vi "Project Omega.vi"() -> ()   [LabVIEW 2020]
uses:
  <vilib>/DAQmx/read.llb/DAQmx Read (Analog 2D DBL NChan NSamp).vi
  <vilib>/DAQmx/create/channels.llb/DAQmx Create Channel (AI-Voltage-Basic).vi
  <vilib>/DAQmx/create/channels.llb/DAQmx Create Channel (AI-Voltage-Custom with Excitation).vi
  <vilib>/DAQmx/configure/timing.llb/DAQmx Timing (Sample Clock).vi
  <vilib>/DAQmx/miscellaneous.llb/DAQmx Fill In Error Info.vi
  <vilib>/Analysis/NI_AALPro.lvlib
panel:
  in  "Path":path
  in  "STOP":bool
  out "Displacement(mm)":dbl[](array[numeric])
  out "Period of Vibration (T)":dbl
  out "Natural Frequency f(n)":dbl
  out "Circular Natural frequency w(n)":dbl
  out "Mass of the spring system(lbm)":dbl
  out "Displacement":dbl
  in  "Displacement offset":dbl
  in  "Load offset":dbl
  out "Force Value (lbf)":dbl
  out "Stiffness of spring(k)":dbl
  out "Load vs Displacement":cluster{dbl[], dbl[]}(graph)
  out "Load vs Time":cluster{dbl[], dbl[]}(graph)
  out "Displacement vs Time":cluster{dbl[], dbl[]}(graph)
  in  "DAQ Rate(Hz)":dbl
  in  "Time to acquire Data(s)":dbl
  in  "Load description":string="Pounds - lbf"
  in  "Displacement custom scale":tag
  in  "Displacement DAQ Channel":tag
  in  "Displacement  Description":string="Positon- inches"
  in  "Load Transducer Scale:":tag
  in  "Load DAQ Channel":tag
  # "DAQ Input"
  # "Results"
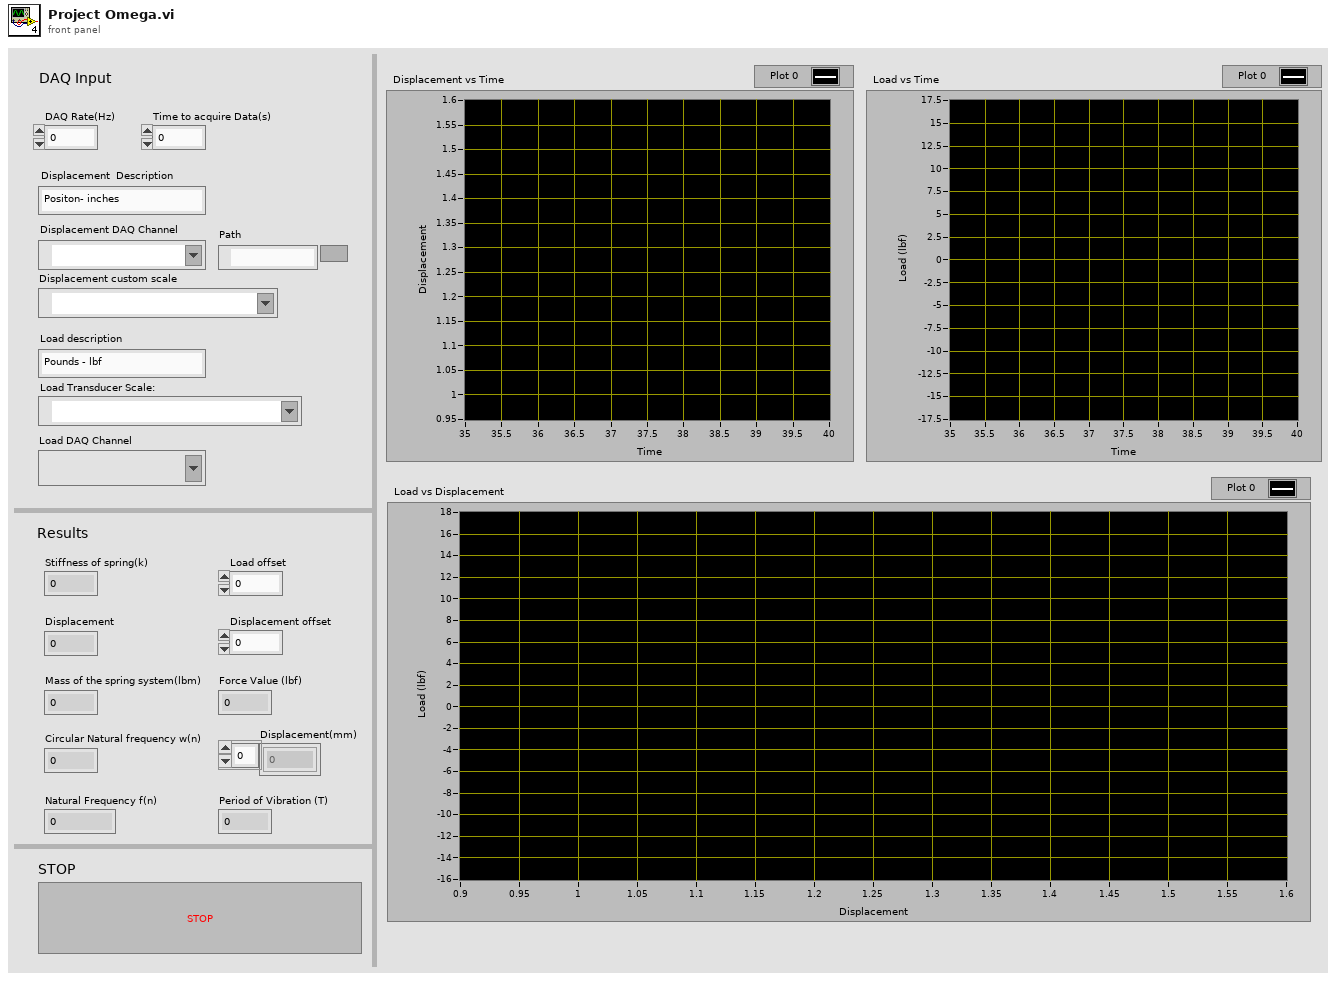
[diagram p1: front panel]
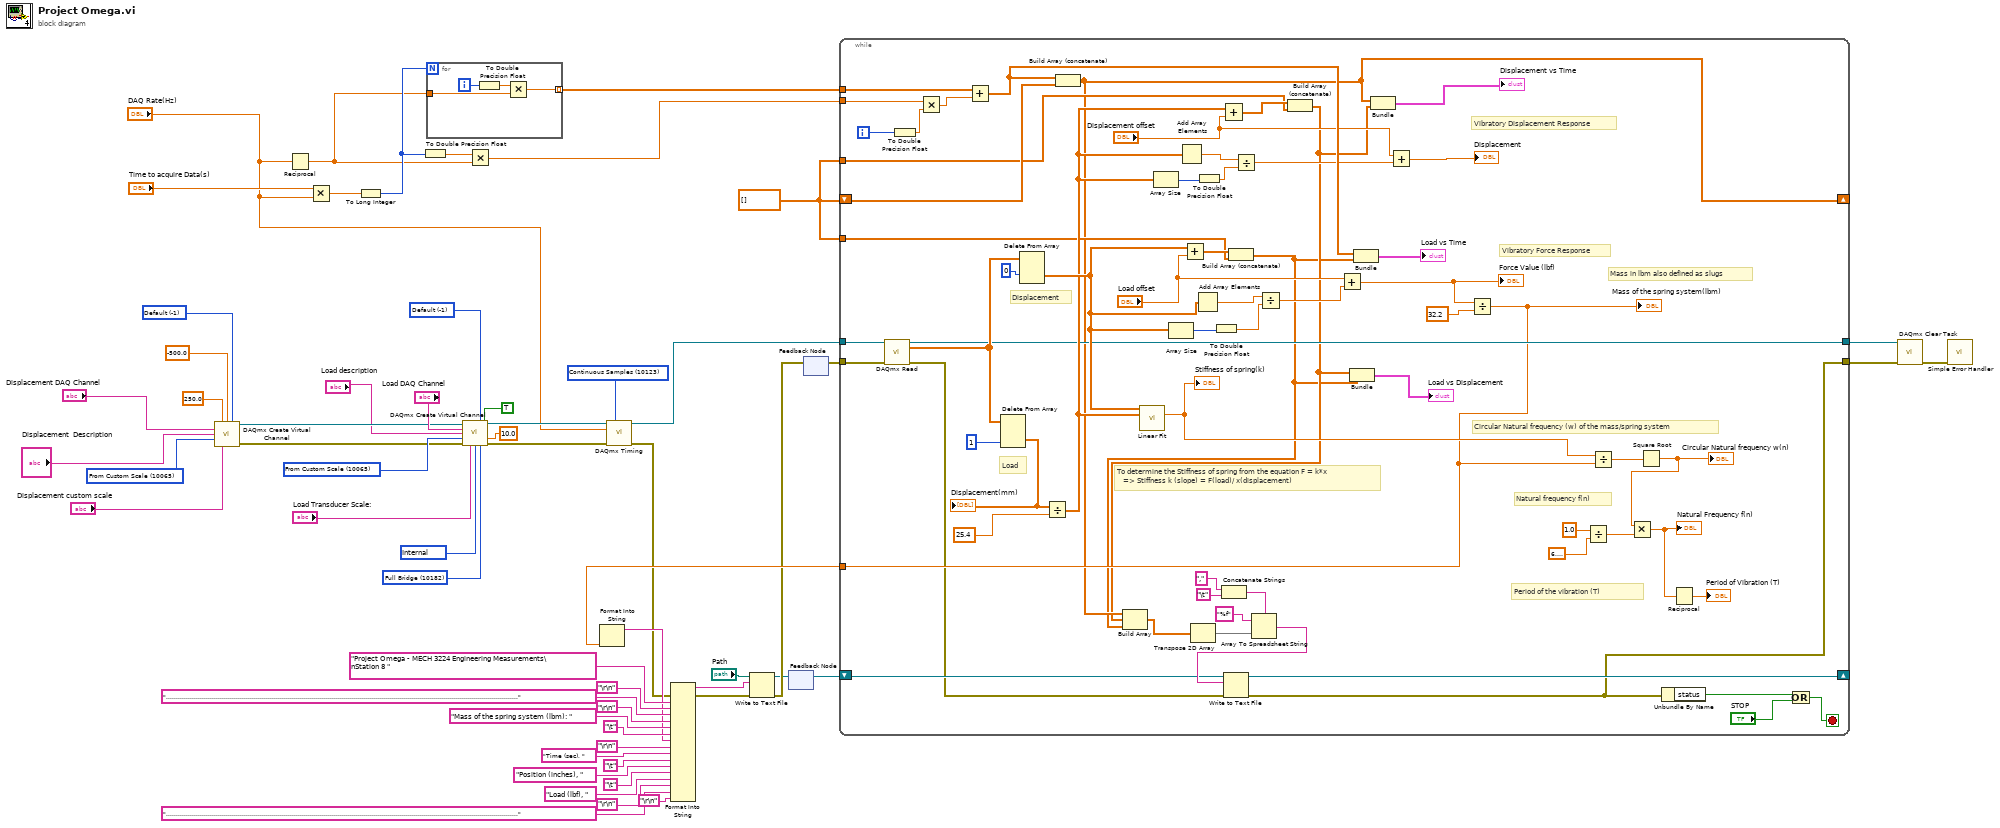
[diagram p0: block diagram]
diagram:
  w3 = dbl[] []
  w43 = 10065 items=["Volts"=10348, "From Custom Scale"=10065] ("units")
  w45 = -1 items=["Default"=-1, "RSE"=10083, "NRSE"=10078, "Differential"=10106, "Pseudodifferential"=12529] ("input terminal configuration")
  w39 = 10182 items=["Full Bridge"=10182, "Half Bridge"=10187, "Quarter Bridge"=10270, "No Bridge"=10228] ("bridge configuration")
  w53 = 10200 items=["Internal"=10200, "External"=10167, "None"=10230] ("voltage excitation source")
  w41 = 10123 items=["Finite Samples"=10178, "Continuous Samples"=10123, "Hardware Timed Single Point"=12522] ("sample mode")
  w55 = 10065 items=["Volts"=10348, "From Custom Scale"=10065] ("units")
  w57 = -1 items=["Default"=-1, "RSE"=10083, "NRSE"=10078, "Differential"=10106, "Pseudodifferential"=12529] ("input terminal configuration")
  n1 = call-poly <vilib>:"DAQmx Create Virtual Channel.vi"("maximum value"=250.0, "minimum value"=-500.0, "input terminal configuration"=w45, "physical channels"="Displacement DAQ Channel", "name to assign"="Displacement  Description", "units"=w43, "custom scale name"="Displacement custom scale") -> ("task out"=w51:refnum<k21>, "error out"=w40:errorcluster)  [unwired: 7 in]
  n2 = Reciprocal(x="DAQ Rate(Hz)") -> (1/x=w34:dbl)
  n3 = Multiply(x="Time to acquire Data(s)", y="DAQ Rate(Hz)") -> (x*y=w37:dbl)
  n4 = To Long Integer(number=w37) -> (32bit integer=w35:i32)
  n5 = To Double Precision Float(number=w35) -> (double precision float=w36:dbl)
  n6 = for {
    N: w35 -> [_]
    tunnel: w34 -> [w61]
    tunnel: [w60] -> w30 mode=indexing
    i -> [w63]
    n7 = To Double Precision Float(number=w63) -> (double precision float=w62:dbl)
    n8 = Multiply(x=w62, y=w61) -> (x*y=w60:dbl)
  }
  n9 = call-poly <vilib>:"DAQmx Create Virtual Channel.vi"("task in"=w51, "input terminal configuration"=w57, "physical channels"="Load DAQ Channel", "use excitation for scaling"=TRUE, "name to assign"="Load description", "units"=w55, "voltage excitation value"=10.0, "error in"=w40, "custom scale name"="Load Transducer Scale:", "voltage excitation source"=w53, "bridge configuration"=w39) -> ("task out"=w58:refnum<k21>, "error out"=w59:errorcluster)  [unwired: 3 in]
  n10 = Multiply(x=w36, y=w34) -> (x*y=w31:dbl)
  n11 = call-poly <vilib>:"DAQmx Timing.vi"("task/channels in"=w58, "sample mode"=w41, "rate"="DAQ Rate(Hz)", "error in"=w59) -> ("task out"=w32:refnum<k21>, "error out"=w8:errorcluster)  [unwired: 10 in]
  n12 = feedback #1() -> (w4:refnum<file>)  [unwired: 1 in]
  n13 = feedback #2() -> (w6:errorcluster)  [unwired: 1 in]
  n14 = while {
    tunnel: w32 -> [w89]
    tunnel: w31 -> [w87]
    tunnel: w30 -> [w86]
    tunnel: [w84] -> w29
    tunnel: [w83] -> w22
    tunnel: w6 -> [w82]
    shift-right: [w67] -> _
    shift-left: w4 -> [w68]
    tunnel: w3 -> [w81]
    shift-right: [w71] -> _
    shift-left: w3 -> [w80]
    tunnel: w3 -> [w79]
    tunnel: [w64] -> w1
    i -> [w88]
    stop <- w90 stop-if-true
    # "Period of the vibration (T)"
    # "Natural frequency f(n)"
    # "Circular Natural frequency (w) of the mass/spring system"
    # "Vibratory Displacement Response"
    # "Vibratory Force Response"
    # "Mass in lbm also defined as slugs"
    # "To determine the Stiffness of spring from the equation F = k*x\n   => Stiffness k (slope) = F(load)/ x(displacement)"
    # "Load"
    # "Displacement"
    n15 = call-poly <vilib>:"DAQmx Read.vi"("task/channels in"=w89, "error in"=w82) -> ("task out"=w84:refnum<k21>, "data"=w126:dbl[][], "error out"=w65:errorcluster)  [unwired: 11 in]
    n16 = To Double Precision Float(number=w88) -> (double precision float=w123:dbl)
    n17 = Multiply(x=w87, y=w123) -> (x*y=w122:dbl)
    n18 = Add(x=w86, y=w122) -> (x+y=w121:dbl[])
    n19 = Delete From Array(array=w126, index (row)=1) -> (deleted portion=w94:dbl[])  [unwired: 2 in, 1 out]
    "Displacement(mm)" <- w94
    n20 = Delete From Array(array=w126, index (row)=0 ("disabled index (col)")) -> (deleted portion=w115:dbl[])  [unwired: 2 in, 1 out]
    n21 = Divide(x=w94, y=25.4 ("Waveform")) -> (x/y=w92:dbl[])
    n22 = Build Array (concatenate)(w121, w80) -> (w71:dbl[])
    n23 = call <vilib>:"Linear Fit.vi"("Y"=w115, "X"=w92) -> ("slope"=w96:dbl)  [unwired: 9 in, 4 out]
    "Stiffness of spring(k)" <- w96
    n24 = Array Size(array=w92) -> (size(s)=w111:i32)
    n25 = Array Size(array=w115) -> (size(s)=w116:i32)
    n26 = Add Array Elements(numeric array=w92) -> (sum=w113:dbl)
    n27 = Add(x=w115, y="Load offset") -> (x+y=w120:dbl[])
    n28 = Add Array Elements(numeric array=w115) -> (sum=w118:dbl)
    n29 = To Double Precision Float(number=w111) -> (double precision float=w112:dbl)
    n30 = To Double Precision Float(number=w116) -> (double precision float=w117:dbl)
    n31 = Add(x=w92, y="Displacement offset") -> (x+y=w110:dbl[])
    n32 = Concatenate Strings("," ("delimiter (Tab)"), "\t") -> (w73:string)
    n33 = Build Array (concatenate)(w120, w81) -> (w69:dbl[])
    n34 = Divide(x=w113, y=w112) -> (x/y=w109:dbl)
    n35 = Divide(x=w118, y=w117) -> (x/y=w114:dbl)
    n36 = Build Array (concatenate)(w110, w79) -> (w70:dbl[])
    n37 = Build Array(w71, w70, w69) -> (w78:dbl[][])
    n38 = Transpose 2D Array(2D array=w78) -> (transposed array=w77:dbl[][])
    n39 = Array To Spreadsheet String(delimiter (Tab)=w73, array=w77, 3:"%f" ("format string")) -> (spreadsheet string=w72:string)
    n40 = Write to Text File(file (use dialog)=w68, text=w72, error in=w65) -> (refnum out=w67:refnum<file>, error out=w64:errorcluster)  [unwired: 1 in, 1 out]
    n41 = Add(x="Load offset", y=w114) -> (x+y=w106:dbl)
    "Force Value (lbf)" <- w106
    n42 = Bundle(w70, w69) -> (→"Load vs Displacement":cluster{dbl[], dbl[]})  [unwired: 1 in]
    n43 = Bundle(w121, w69) -> (→"Load vs Time":cluster{dbl[], dbl[]})  [unwired: 1 in]
    n44 = Bundle(w71, w70) -> (→"Displacement vs Time":cluster{dbl[], dbl[]})  [unwired: 1 in]
    n45 = Add(x="Displacement offset", y=w109) -> (x+y=→"Displacement":dbl)
    n46 = Divide(x=w106, y=32.2) -> (x/y=w83:dbl)
    "Mass of the spring system(lbm)" <- w83
    n47 = Divide(x=1.0, y=6.283185307179586) -> (x/y=w100:dbl)
    n48 = Divide(x=w96, y=w83) -> (x/y=w103:dbl)
    n49 = Square Root(x=w103) -> (sqrt(x)=w99:dbl)
    "Circular Natural frequency w(n)" <- w99
    n50 = Multiply(x=w99, y=w100) -> (x*y=w98:dbl)
    "Natural Frequency f(n)" <- w98
    n51 = Unbundle By Name(w64) -> ("status"=w66:bool)
    n52 = Reciprocal(x=w98) -> (1/x=→"Period of Vibration (T)":dbl)
    n53 = Or(x=w66, y="STOP") -> (x .or. y?=w90:bool)
  }
  n54 = Format Into String(w22) -> (resulting string=w18:string)  [unwired: 3 in, 1 out]
  n55 = Format Into String(error in=w8, "Project Omega - MECH 3224 Engineering Measurements\nStation 8 ", "\r\n", "................................................................................................................................................................................", "\r\n", "Mass of the spring system (lbm): ", "\t", w18, "\r\n", "Time (sec), ", "\t", "Position (inches), ", "\t", "Load (lbf), ", "\r\n", "................................................................................................................................................................................", "\r\n") -> (resulting string=w2:string, error out=w21:errorcluster)  [unwired: 2 in]
  n56 = Write to Text File(file (use dialog)="Path", text=w2, error in=w21) -> (refnum out=w5:refnum<file>, error out=w7:errorcluster)  [unwired: 1 in, 1 out]
  n57 = feedback-in #1(w5) -> ()
  n58 = feedback-in #2(w7) -> ()
  n59 = call <vilib>:"DAQmx Clear Task.vi"("task in"=w29, "error in"=w1) -> ("error out"=w28:errorcluster)  [unwired: 13 in]
  n60 = call <vilib>:"Simple Error Handler.vi"("error in (no error)"=w28) -> ()  [unwired: 4 in, 5 out]
